vi "Set Level.vi"(8 "error in (no error)":errorcluster, 10 "Setpoint":dbl min=0.0 max=16.0 step=0.5 format="%04.1f", 11 "SS P100 Settings In":T1) -> (0 "error out":errorcluster, 1 "Connection Error":bool, 3 "SS P100 Settings Out":T1)   [LabVIEW 2018, in "Sonic Systems P100.lvlib"]
uses:
  Sonic Systems P100.lvlib
  Sonic Systems P100 Settings.ctl
  support/Support Library.lvlib
panel:
  out "read buffer 2":string
  out "read buffer":string
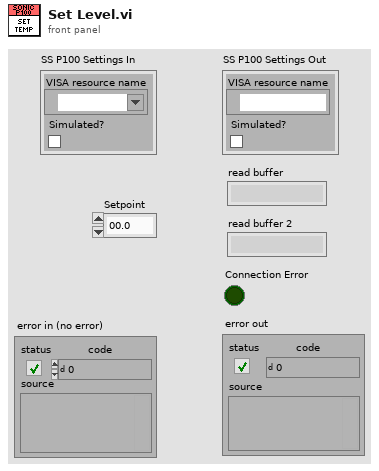
[diagram p1: front panel]
types:
  T1 = typedef "Sonic Systems P100.lvlib/Sonic Systems P100 Settings.ctl" = cluster{"VISA resource name":refnum<visa-resource-name>, "Simulated?":bool}
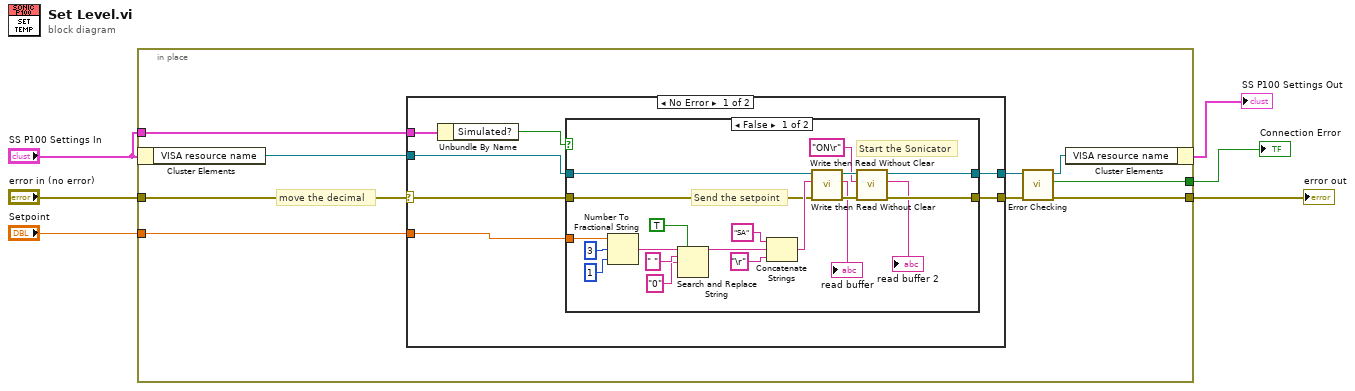
[diagram p0: block diagram]
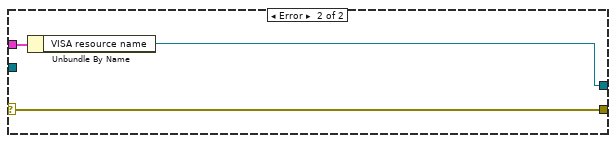
[diagram p3: hidden frame]
diagram:
  n1 = in-place {
    in-place-border: "error in (no error)" -> [w15]
    in-place-border: "SS P100 Settings In" -> [w12]
    in-place-border: [w11] -> w5
    in-place-border: [w10] -> w4
    in-place-border: "Setpoint" -> [w7]
    # "move the decimal"
    n2 = in-place-cluster #1("SS P100 Settings In") -> ("VISA resource name"=w9:refnum<visa-resource-name>)
    n3 = case shown="No Error" w15 {
      selector: w15 -> [w22 w47]
      tunnel: w12 -> [w18 w46]
      tunnel: [w21 w47] -> w13
      tunnel: [w20 w45] -> w14
      tunnel: w7 -> [w17 _]
      tunnel: w9 -> [w16 _]
      frame No Error {
        n4 = Unbundle By Name(w18) -> ("Simulated?"=w19:bool)
        n5 = case shown="False" w19 {
          tunnel: w22 -> [w30 w44]
          tunnel: [w25 w44] -> w21
          tunnel: [w26 w43] -> w20
          tunnel: w16 -> [w32 w43]
          tunnel: w17 -> [w40 _]
          frame False {
            # "Start the Sonicator"
            # "Send the setpoint"
            n6 = Number To Fractional String(number=w40, width (-)=i16 3, precision (6)=i16 1) -> (F-format string=w34:string)  [unwired: 1 in]
            n7 = Search and Replace String(replace all?=TRUE ("replace all? (F)"), input string=w34, search string=" ", replace string="0" ("replace string (\"\")")) -> (result string=w33:string)  [unwired: 4 in, 3 out]
            n8 = Concatenate Strings("SA" ("string"), w33, "\r" ("string")) -> (w31:string)
            n9 = call "Write then Read Without Clear.vi"("error in"=w30, "write buffer"=w31, "VISA resource name in"=w32) -> ("error out"=w28:errorcluster, "read buffer"=→"read buffer":string, "VISA resource name out"=w29:refnum<visa-resource-name>)  [unwired: 5 in, 1 out]
            n10 = call "Write then Read Without Clear.vi"("error in"=w28, "write buffer"="ON\r", "VISA resource name in"=w29) -> ("error out"=w25:errorcluster, "read buffer"=→"read buffer 2":string, "VISA resource name out"=w26:refnum<visa-resource-name>)  [unwired: 5 in, 1 out]
          }
          frame True {
          }
        }
      }
      frame Error {
        n11 = Unbundle By Name(w46) -> ("VISA resource name"=w45:refnum<visa-resource-name>)
      }
    }
    n12 = call "Error Checking.vi"("error in (no error)"=w13, "VISA resource name"=w14) -> ("error out"=w10:errorcluster, "Connection Error"=w11:bool, "VISA resource name"=w8:refnum<visa-resource-name>)  [unwired: 7 in]
    n13 = in-place-cluster #1("VISA resource name"=w8) -> (→"SS P100 Settings Out":T1)
  }
  "error out" <- w4
  "Connection Error" <- w5
